vi "SRA_FINAL.vi"() -> ()   [LabVIEW 2022 SP3]
uses:
  class/mqtt/mqttTypedef/mqttSubscribeCluster.ctl
  class/mqtt/mqttTypedef/mqttQOSlevel.ctl
  class/mqtt/mqttTypedef/mqttBroker.ctl
  class/mqtt/mqttTypedef/mqttWillInformation.ctl
  class/mqtt/mqttTXqueue/mqttTXdataQueueFunction.ctl
  class/mqtt/mqttConfigFunction.ctl
  class/mqtt/mqttTXqueue/mqttRXsubscriptionEventFunction.ctl
  class/mqtt/mqttTypedef/mqttConnectionMeta.ctl
  <vilib>/Instr/_visa.llb/VISA Configure Serial Port (Instr).vi
  class/mqtt/mqtt.lvclass
panel:
  in  "stop":bool
  out "quit":bool
  in  "?":enum32{"HMI", "MQTT"}(tab)=enum."MQTT"
  in  "Message Arduino - Angles":bool
  out "Angles_Review":string
  in  "Message Arduino -  Mode":bool
  in  "Byte":u32
  out "Read Target":string
  out "Number_of_runs":i16
  in  "Joint 1":u8(knob) scale=40.0..140.0
  in  "Claw":bool
  in  "Buttom":u8(knob) scale=50.0..150.0
  in  "Joint 2":u8(knob) scale=45.0..100.0
  out "Applied Mode":string
  out "Running":bool
  out "Stopped":bool
  out "RX Mode":string
  out "valueSent":string
  in  "Enable Auto Publish":bool
  in  "subscribe":bool
  in  "topic":string="/v1.6/devices/arduino-sra/Number_of_runs"
  out "publishSuccess":bool
  out "subscribeSuccess":bool
  in  "subscriptionInfo":T1[](array[typedef])=[{"Topic"="/v1.6/devices/arduino/VAR_NAME/lv", "QoS"=enum."At least once"}]
  in  "connect":bool
  in  "disconnect":bool
  out "RX Topic":string
  out "RX Value":string
  in  "publish":bool
  out "value":string="0"
  out "autoPublish":bool
  in  "broker":T3={"address"="industrial.api.ubidots.com", "port"=1883, "connTimeout"=30000, "writeTimeout"=2000, "readTimeout"=2000, "subTimeout"=300000}
  in  "client":string="SMRTTECH3CC3-SRA"
  in  "User Info":T4={"User Name"="BBFF-Kf0hC2lkCnUdX4fIyr863pX9wMI0EG", "Password"=""}
  # "Smart Robotic Arm Control Panel"
  # "Automatic Mode"
  # "Select Mode"
  # "Hybrid Mode"
  # "[50° - 150°]"
  # "[40° - 140°]"
  # "Set Byte to 3  for Automatic mode\nOrtherwise set it to 0"
  # "0.0 - Manual\n             1.0 - Hybrid\n             2.0 - Automatic"
  # "[45° - 100°]"
  # "Open(0)"
  # "Close(1)"
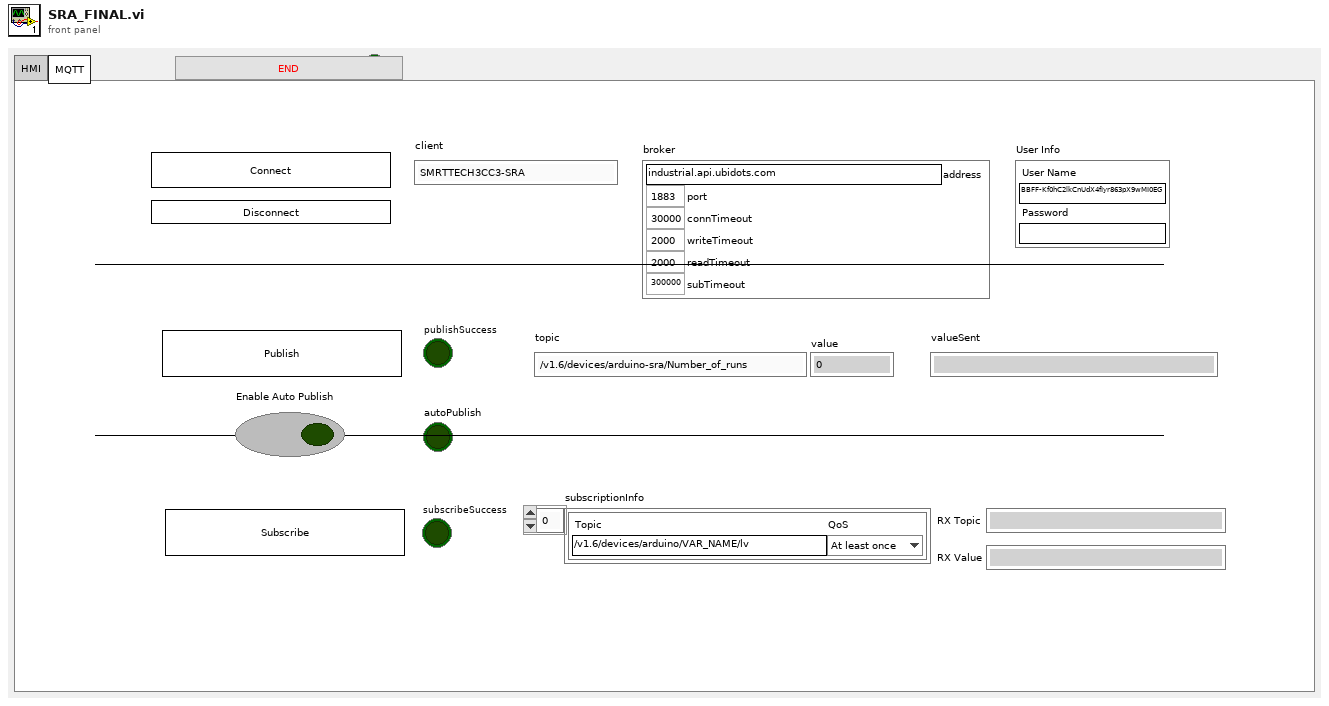
[diagram p1: front panel]
types:
  T1 = typedef "mqttSubscribeCluster.ctl" = cluster{"Topic":string, "QoS":T2}
  T2 = typedef "mqttQOSlevel.ctl" = enum8{"At most once", "At least once", "Exactly once", "Reserved"}
  T3 = typedef "mqttBroker.ctl" = cluster{"address":string, "port":u16, "connTimeout":i32, "writeTimeout":i32, "readTimeout":i32, "subTimeout":i32}
  T4 = typedef "mqttWillInformation.ctl" = cluster{"User Name":string, "Password":string}
  T5 = typedef "mqttRXsubscriptionEventFunction.ctl" = enum16{"init", "deinit", "getEventRef", "event"}
  T6 = typedef "mqtt.lvclass/mqttConfigFunction.ctl" = enum16{"init", "deinit", "set", "get"}
  T7 = typedef "mqttTXdataQueueFunction.ctl" = enum16{"init", "deinit", "getQueue", "enqueue"}
  T8 = enum8{"Enabled", "Disabled", "Disabled and Grayed Out"}
  T9 = typedef "mqttConnectionMeta.ctl" = cluster{"retain":bool, "duplicate":bool, "qos":T2}
  T10 = typedef "mqttConnectionStatus.ctl" = enum16{"Connection accepted", "Connection refused: unacceptable protocol version", "Connection refused: identifier rejected", "Connection refused: Server unavailable", "Connection refused: bad user name or password", "Connection refused: not authorized"}
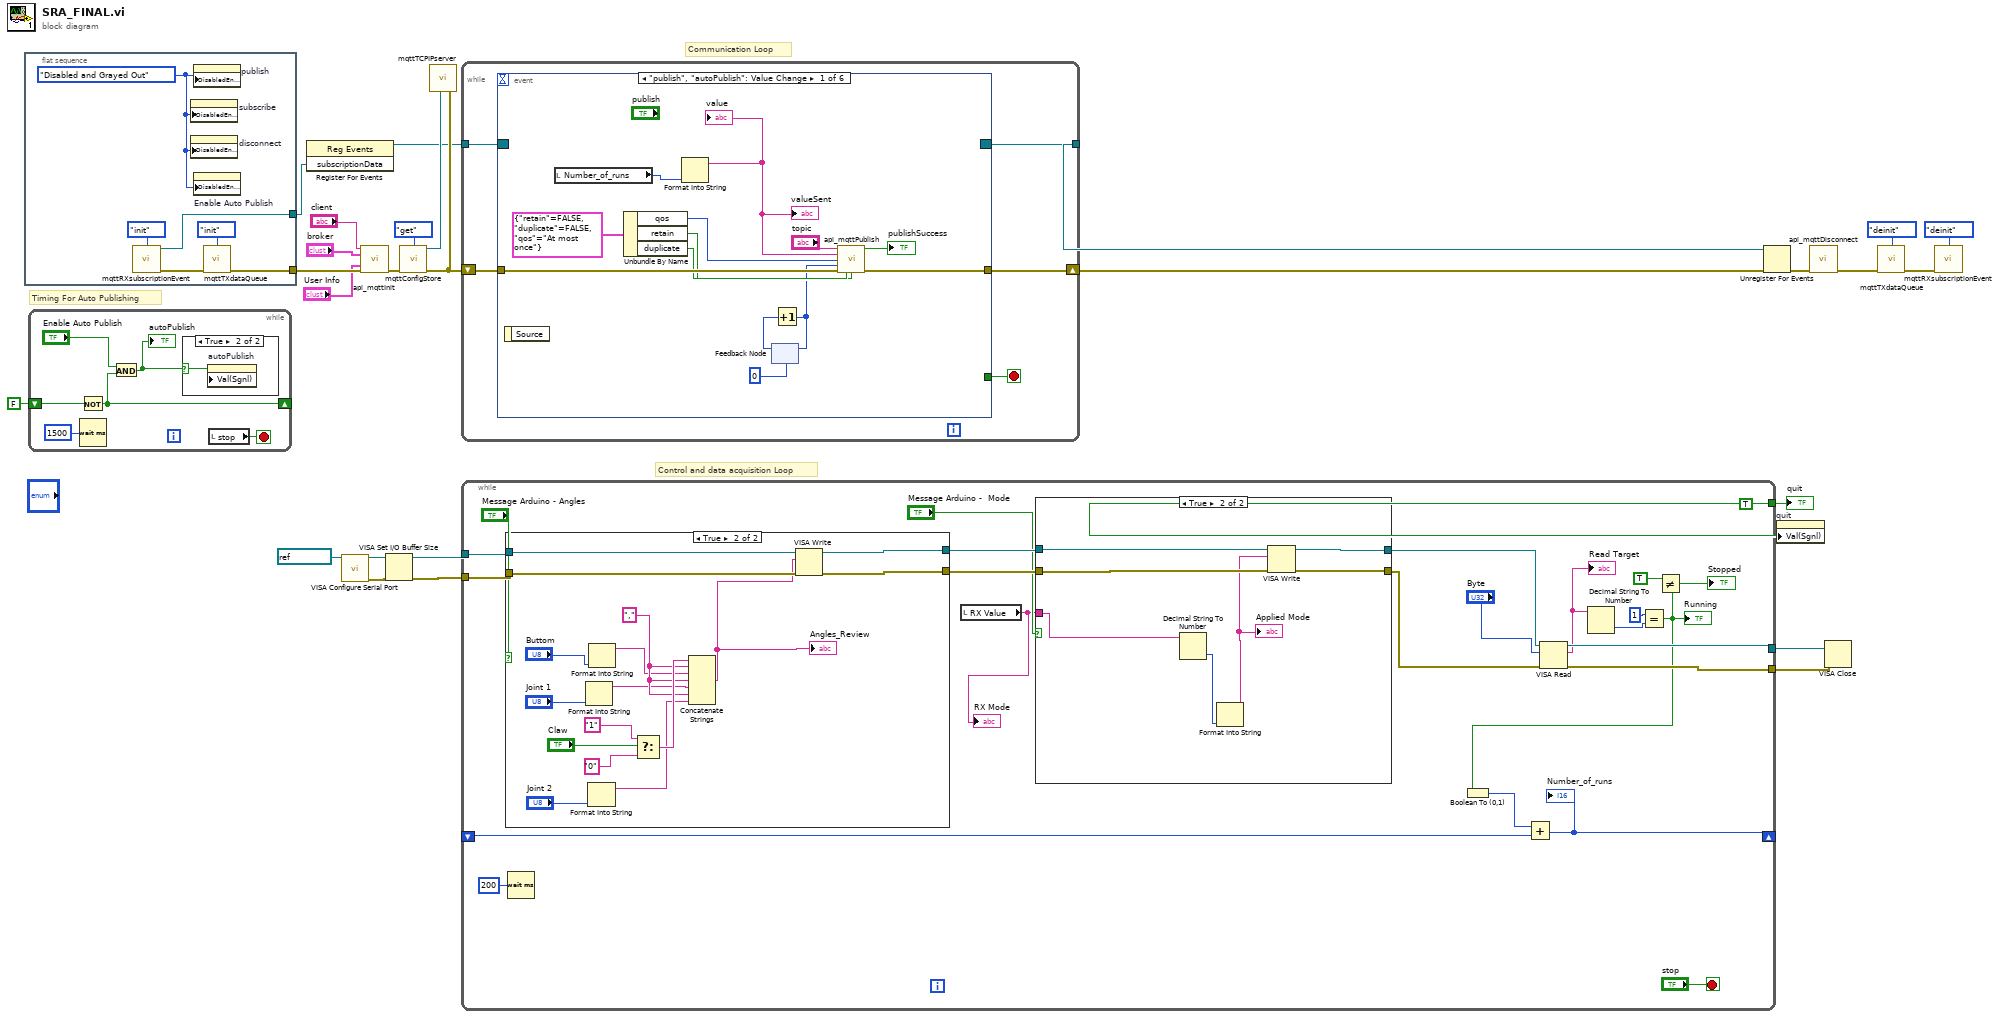
[diagram p0: block diagram]
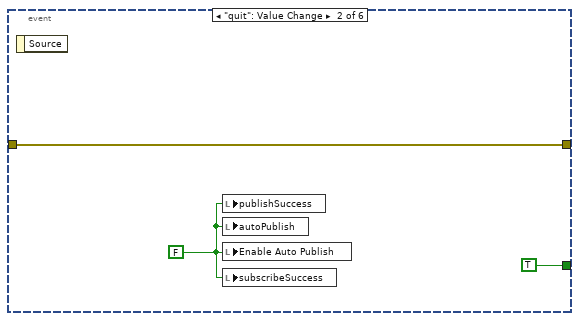
[diagram p5: hidden frame]
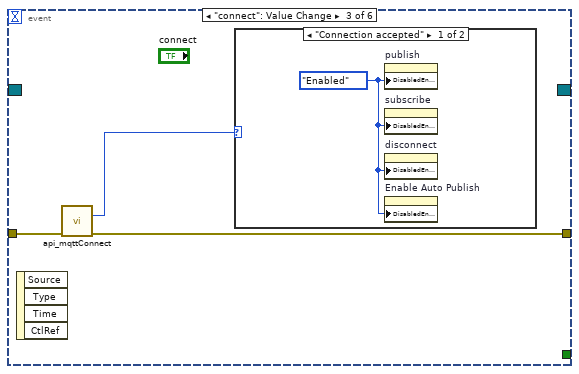
[diagram p6: hidden frame]
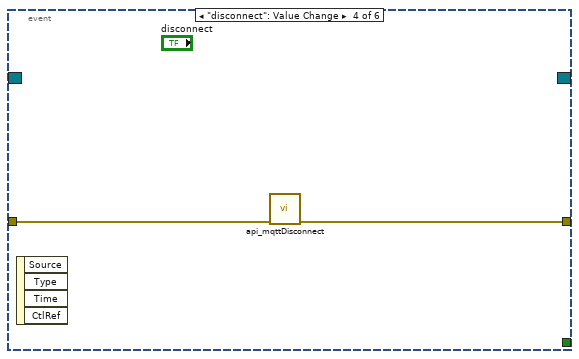
[diagram p8: hidden frame]
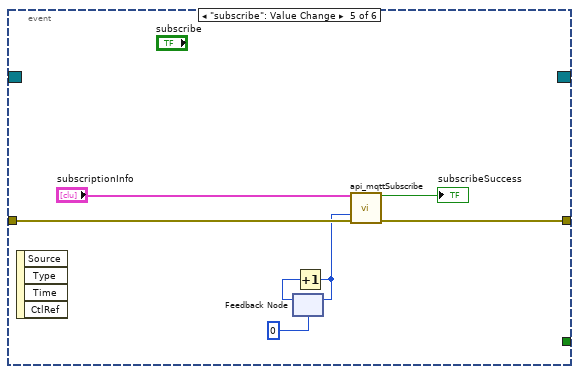
[diagram p9: hidden frame]
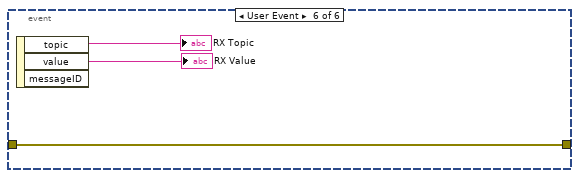
[diagram p10: hidden frame]
diagram:
  # "Timing For Auto Publishing"
  # "Control and data acquisition Loop"
  # "Communication Loop"
  n1 = flat-sequence {
    tunnel: [w31] -> w25
    tunnel: [w28] -> w19
    frame #0 {
      w27 = T8."Disabled and Grayed Out" ("Disabled")
      n2 = call "mqttRXsubscriptionEvent.vi"("function"=mqttRXsubscriptionEventFunction."init") -> ("subscriptionData"=w28:refnum<user-event>, "error out"=w30:errorcluster)  [unwired: 13 in]
      n3 = property on="subscribe" class="Bool"("DisabledEnum"=w27) -> ()  [unwired: 2 in, 2 out]
      n4 = property on="disconnect" class="Bool"("DisabledEnum"=w27) -> ()  [unwired: 2 in, 2 out]
      n5 = property on="publish" class="Bool"("DisabledEnum"=w27) -> ()  [unwired: 2 in, 2 out]
      n6 = property on="Enable Auto Publish" class="Bool (strict)"("DisabledEnum"=w27) -> ()  [unwired: 2 in, 2 out]
      n7 = call "mqttTXdataQueue.vi"("function"=mqttTXdataQueueFunction."init", "error in (no error)"=w30) -> ("error out"=w31:errorcluster)  [unwired: 12 in, 1 out]
    }
  }
  n8 = while {
    shift-right: [w33] -> _
    shift-left: FALSE -> [w34]
    stop <- w36 stop-if-true
    n9 = Not(x=w34) -> (.not. x?=w33:bool)
    n10 = Wait (ms)(milliseconds to wait=u32 1500) -> ()  [unwired: 1 out]
    n11 = And(x="Enable Auto Publish", y=w33) -> (x .and. y?=w35:bool)
    "autoPublish" <- w35
    n12 = case shown="True" w35 {
      selector: w35 -> [_ w39]
      frame False {
      }
      frame True {
        n13 = property on="autoPublish" class="Bool"("Val(Sgnl)"=w39) -> ()  [unwired: 2 in, 2 out]
      }
    }
    n14 = local read "stop"() -> (w36:bool)
  }
  n15 = register-events(w19) -> (reference out=w18:refnum<event-registration>)  [unwired: 2 in, 1 out]
  n16 = call-poly "VISA Configure Serial Port"("VISA resource name"=refnum<visa-resource-name> "COM5") -> ("VISA resource name out"=w6:refnum<visa-resource-name>, "error out"=w5:errorcluster)  [unwired: 13 in]
  n17 = call "api_mqttInit.vi"("client"="client", "broker"="broker", "User Info"="User Info", "error in (no error)"=w25) -> ("error out"=w23:errorcluster)  [unwired: 11 in]
  n18 = VISA Set I/O Buffer Size(VISA resource name=w6, error in (no error)=w5) -> (VISA resource name out=w3:refnum<visa-resource-name>, error out=w4:errorcluster)  [unwired: 2 in]
  n19 = call "mqttConfigStore.vi"("function"=mqttConfigFunction."get", "error in (no error)"=w23) -> ("mqtt.lvclass out"=w22:refnum<class "mqtt.lvclass">, "error out"=w21:errorcluster)  [unwired: 12 in]
  n20 = call "mqttTCPIPserver.vi"("mqtt.lvclass"=w22, "error in (no error)"=w21) -> ()  [unwired: 12 in, 2 out]
  n21 = while {
    tunnel: [TRUE] -> w8
    tunnel: w3 -> [w56]
    tunnel: [w61] -> w2
    tunnel: [w60] -> w1
    tunnel: w4 -> [w55]
    shift-right: [w58] -> _
    shift-left: _ -> [w57]
    stop <- "stop" stop-if-true
    n22 = case shown="True" "Message Arduino - Angles" {
      tunnel: [w74 w90] -> w53
      tunnel: [w73 w89] -> w52
      tunnel: w56 -> [w74 w88]
      tunnel: w55 -> [w73 w85]
      frame False {
      }
      frame True {
        w82 = ","
        n23 = Format Into String("Joint 1") -> (resulting string=w77:string)  [unwired: 3 in, 1 out]
        n24 = Format Into String("Joint 2") -> (resulting string=w76:string)  [unwired: 3 in, 1 out]
        n25 = Format Into String("Buttom") -> (resulting string=w80:string)  [unwired: 3 in, 1 out]
        n26 = Select(t="1", s="Claw", f="0") -> (s? t:f=w84:string)
        n27 = Concatenate Strings(w84, w82, w80, w82, w77, w82, w76) -> (w75:string)
        "Angles_Review" <- w75
        n28 = VISA Write(VISA resource name=w88, write buffer=w75, error in (no error)=w85) -> (VISA resource name out=w90:refnum<visa-resource-name>, error out=w89:errorcluster)  [unwired: 1 out]
      }
    }
    n29 = Wait (ms)(milliseconds to wait=u32 200) -> ()  [unwired: 1 out]
    n30 = local read "RX Value"() -> (w40:string)
    "RX Mode" <- w40
    n31 = case shown="True" "Message Arduino -  Mode" {
      tunnel: w53 -> [w65 w72]
      tunnel: w52 -> [w64 w69]
      tunnel: [w65 w71] -> w51
      tunnel: [w64 w70] -> w50
      tunnel: w40 -> [_ w66]
      frame False {
      }
      frame True {
        n32 = Decimal String To Number(string=w66) -> (number=w67:i32)  [unwired: 2 in, 1 out]
        n33 = Format Into String(w67) -> (resulting string=w68:string)  [unwired: 3 in, 1 out]
        "Applied Mode" <- w68
        n34 = VISA Write(VISA resource name=w72, write buffer=w68, error in (no error)=w69) -> (VISA resource name out=w71:refnum<visa-resource-name>, error out=w70:errorcluster)  [unwired: 1 out]
      }
    }
    n35 = VISA Read(VISA resource name=w51, byte count="Byte", error in (no error)=w50) -> (VISA resource name out=w61:refnum<visa-resource-name>, read buffer=w42:string, error out=w60:errorcluster)  [unwired: 1 out]
    "Read Target" <- w42
    n36 = Decimal String To Number(string=w42) -> (number=w47:i32)  [unwired: 2 in, 1 out]
    n37 = Equal?(x=1, y=w47) -> (x = y?=w41:bool)
    "Running" <- w41
    n38 = Boolean To (0,1)(Boolean=w41) -> (0, 1=w49:i16)
    n39 = Add(x=w49, y=w57) -> (x+y=w58:i16)
    "Number_of_runs" <- w58
    n40 = Not Equal?(x=TRUE, y=w41) -> (x != y?=→"Stopped":bool)
  }
  "quit" <- w8
  n41 = while {
    shift-right: [w95] -> w15
    shift-left: w21 -> [w94]
    tunnel: w18 -> [w92]
    tunnel: [w91] -> w13
    stop <- w93 stop-if-true
    n42 = event shown="[0] \"publish\", \"autoPublish\": Value Change" {
      selector: w92 -> [_ _ _ _ _ _]
      dyn-events: [_ _ _ _ _ _] -> w91
      timeout: _ -> [_ _ _ _ _ _]
      tunnel: [w107 w110 w113 w116 w122 w127] -> w95
      tunnel: w94 -> [w108 w110 w114 w117 w121 w127]
      tunnel: [_ TRUE _ _ _ _] -> w93
      event "publish", "autoPublish": Value Change {
        n43 = event-data() -> ()  [unwired: 1 in, 1 out]
        n44 = local read "Number_of_runs"() -> (w96:i16)
        n45 = Unbundle By Name(T9 {"retain"=FALSE, "duplicate"=FALSE, "qos"=enum."At most once"} ("connMeta")) -> ("qos"=w103:T2, "retain"=w102:bool, "duplicate"=w101:bool)
        n46 = Format Into String(w96) -> (resulting string=w97:string)  [unwired: 3 in, 1 out]
        "value" <- w97
        "valueSent" <- w97
        n47 = feedback #1(u16 0) -> (w99:u16)
        n48 = Increment(x=w99) -> (x+1=w98:u16)
        n49 = feedback-in #1(w98) -> ()
        n50 = call "api_mqttPublish.vi"("topic"="topic", "value"=w97, "QoS (At most once)"=w103, "messageID"=w98, "error in (no error)"=w108, "retain(F)"=w102, "duplicate(F)"=w101) -> ("success"=→"publishSuccess":bool, "error out"=w107:errorcluster)  [unwired: 7 in]
      }
      event "quit": Value Change {
        w109 = FALSE ("Enable Auto Publish")
        n51 = event-data() -> ()  [unwired: 1 in, 1 out]
        n52 = local write "publishSuccess"(w109) -> ()
        n53 = local write "autoPublish"(w109) -> ()
        n54 = local write "Enable Auto Publish"(w109) -> ()
        n55 = local write "subscribeSuccess"(w109) -> ()
      }
      event "connect": Value Change {
        n56 = event-data() -> ()  [unwired: 1 in, 4 out]
        n57 = call "api_mqttConnect.vi"("error in (no error)"=w114) -> ("connStatus"=w112:T10, "error out"=w113:errorcluster)  [unwired: 11 in, 2 out]
        n58 = case shown="\"Connection accepted\"" w112 {
          frame "Connection accepted" {
            w115 = T8."Enabled" ("Disabled")
            n59 = property on="publish" class="Bool"("DisabledEnum"=w115) -> ()  [unwired: 2 in, 2 out]
            n60 = property on="subscribe" class="Bool"("DisabledEnum"=w115) -> ()  [unwired: 2 in, 2 out]
            n61 = property on="disconnect" class="Bool"("DisabledEnum"=w115) -> ()  [unwired: 2 in, 2 out]
            n62 = property on="Enable Auto Publish" class="Bool (strict)"("DisabledEnum"=w115) -> ()  [unwired: 2 in, 2 out]
          }
          frame Default {
          }
        }
      }
      event "disconnect": Value Change {
        n63 = event-data() -> ()  [unwired: 1 in, 4 out]
        n64 = call "api_mqttDisconnect.vi"("error in (no error)"=w117) -> ("error out"=w116:errorcluster)  [unwired: 13 in, 1 out]
      }
      event "subscribe": Value Change {
        n65 = event-data() -> ()  [unwired: 1 in, 4 out]
        n66 = feedback #2(u16 0) -> (w119:u16)
        n67 = Increment(x=w119) -> (x+1=w118:u16)
        n68 = feedback-in #2(w118) -> ()
        n69 = call "api_mqttSubscribe.vi"("subscriptionInfo"="subscriptionInfo", "messageID"=w118, "error in (no error)"=w121) -> ("success"=→"subscribeSuccess":bool, "error out"=w122:errorcluster)  [unwired: 11 in]
      }
      event User Event {
        n70 = event-data() -> ("topic"=→"RX Topic":string, "value"=→"RX Value":string)  [unwired: 1 in, 1 out]
      }
    }
  }
  n71 = Unregister For Events(event registration refnum=w13, error in=w15) -> (error out=w14:errorcluster)
  n72 = property on="quit" class="Bool"("Val(Sgnl)"=w8) -> ()  [unwired: 2 in, 2 out]
  n73 = call "api_mqttDisconnect.vi"("error in (no error)"=w14) -> ("error out"=w20:errorcluster)  [unwired: 13 in, 1 out]
  n74 = VISA Close(VISA resource name=w2, error in (no error)=w1) -> ()  [unwired: 1 out]
  n75 = call "mqttTXdataQueue.vi"("function"=mqttTXdataQueueFunction."deinit", "error in (no error)"=w20) -> ("error out"=w16:errorcluster)  [unwired: 12 in, 1 out]
  n76 = call "mqttRXsubscriptionEvent.vi"("function"=mqttRXsubscriptionEventFunction."deinit", "error in (no error)"=w16) -> ()  [unwired: 12 in, 2 out]
